vi "Amplifier Control.vi"() -> ()   [LabVIEW 2012]
uses:
  <vilib>/DAQmx/write.llb/DAQmx Write (Digital 1D Bool NChan 1Samp 1Line).vi
  <vilib>/DAQmx/miscellaneous.llb/DAQmx Fill In Error Info.vi
panel:
  in  "Switch to Amplifier\n      Offline / Online\n           <--              -->":bool
  in  "stop":bool
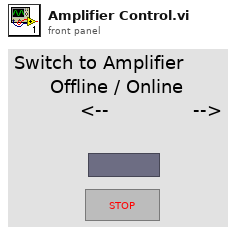
[diagram p1: front panel]
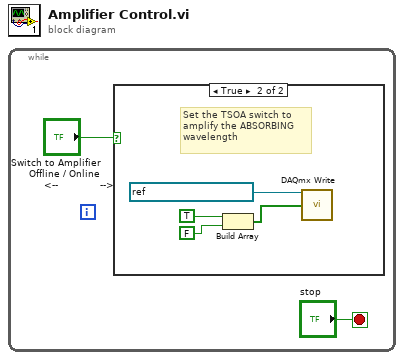
[diagram p0: block diagram]
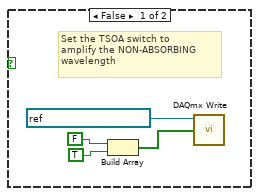
[diagram p2: hidden frame]
diagram:
  n1 = while {
    stop <- "stop" stop-if-true
    n2 = case shown="True" "Switch to Amplifier\n      Offline / Online\n           <--              -->" {
      frame False {
        # "Set the TSOA switch to\namplify the NON-ABSORBING\nwavelength"
        n3 = Build Array(FALSE ("Boolean"), TRUE ("element")) -> (w4:bool[])
        n4 = call-poly <vilib>:"DAQmx Write.vi"("task/channels in"=refnum<k21> "SigToAmpControl", "data"=w4) -> ()  [unwired: 11 in, 3 out]
      }
      frame True {
        # "Set the TSOA switch to\namplify the ABSORBING\nwavelength"
        n5 = Build Array(TRUE ("Boolean"), FALSE ("element")) -> (w8:bool[])
        n6 = call-poly <vilib>:"DAQmx Write.vi"("task/channels in"=refnum<k21> "SigToAmpControl", "data"=w8) -> ()  [unwired: 11 in, 3 out]
      }
    }
  }
